vi "test_marcel.vi"() -> ()   [LabVIEW 2012]
uses:
  OLD_apparatus_VI/VI/Clearing_mode.ctl
  OLD_apparatus_VI/VI/Readout_mode.ctl
  OLD_apparatus_VI/VI/ADC_gain.ctl
  OLD_apparatus_VI/VI/Image_type.ctl
panel:
  out "Numeric":i32
  out "Data type":u32
  in  "Image type":T1=6 items=["8 bit signed"=1, "16 bit signed"=2, "32 bit signed"=3, "32 bit floating"=4, "64 bit floating"=5, "8 bit unsigned"=6, "16 bit unsigned"=7, "32 bit unsigned"=8]
  in  "Number of Images":u32=1000
  in  "Acquire / Focus Flag":u32=1
  in  "stop":bool=TRUE
  out "Number of Cameras":i32
  out "img":sgl[][](graph)
  out "Ydim":u32
  out "Xdim":u32
  out "Camera Handle":u32
  out "error out":errorcluster
  out "Image Handle":u32
  in  "ADC Gain":T2=-1 items=["Use current ADC"=-1, "Use the fastest ADC"=-2, "Use the slowest ADC"=-3]
  in  "ReadoutMode":T3=2.0 caption="Readout Mode" items=["Normal readout"=1.0, "Frame transfer readout"=2.0, "MPP readout"=3.0, "Frame transfer MPP"=4.0, "Alternate timing for normal readout"=5.0, "Alternate timing for frame transfer"=6.0, "Alternate timing for MPP"=7.0, "Alternate timing for frame transfer MPP"=8.0, "Interline"=9.0]
  in  "ClearMode":T4=1.0 caption="Clearing Mode" items=["Clear never"=1.0, "Clear pre-exposure"=2.0, "Clear pre-sequence"=3.0, "Clear post-sequence"=4.0, "Clear pre- and post-sequence"=5.0, "Clear pre-exposure and post-sequence"=6.0]
  in  "EMGain":dbl=3500.0 caption="EM Gain" format="%.2f"
  in  "Exposure (sec)":dbl=0.01 format="%.3f"
  in  "Temperature":dbl=-70.0 format="%.2f"
  in  "error in (no error)":errorcluster
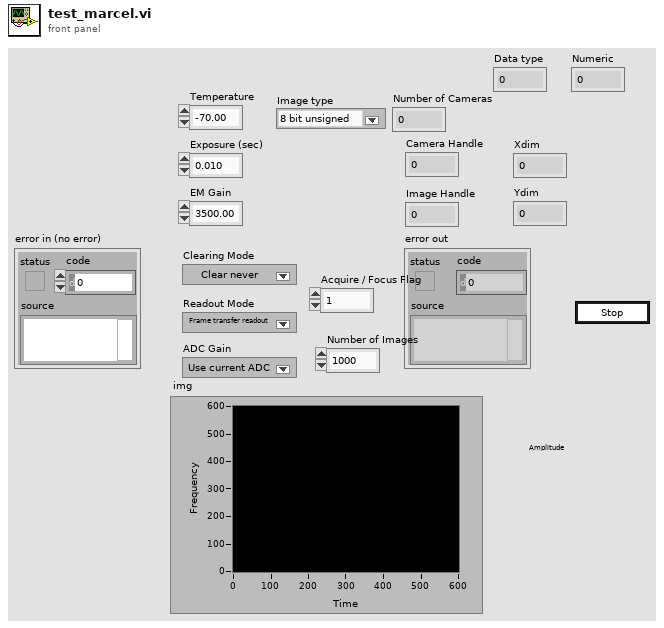
[diagram p1: front panel]
types:
  T1 = typedef "Image_type.ctl" = u32
  T2 = typedef "ADC_gain.ctl" = i32
  T3 = typedef "Readout_mode.ctl" = dbl
  T4 = typedef "Clearing_mode.ctl" = dbl
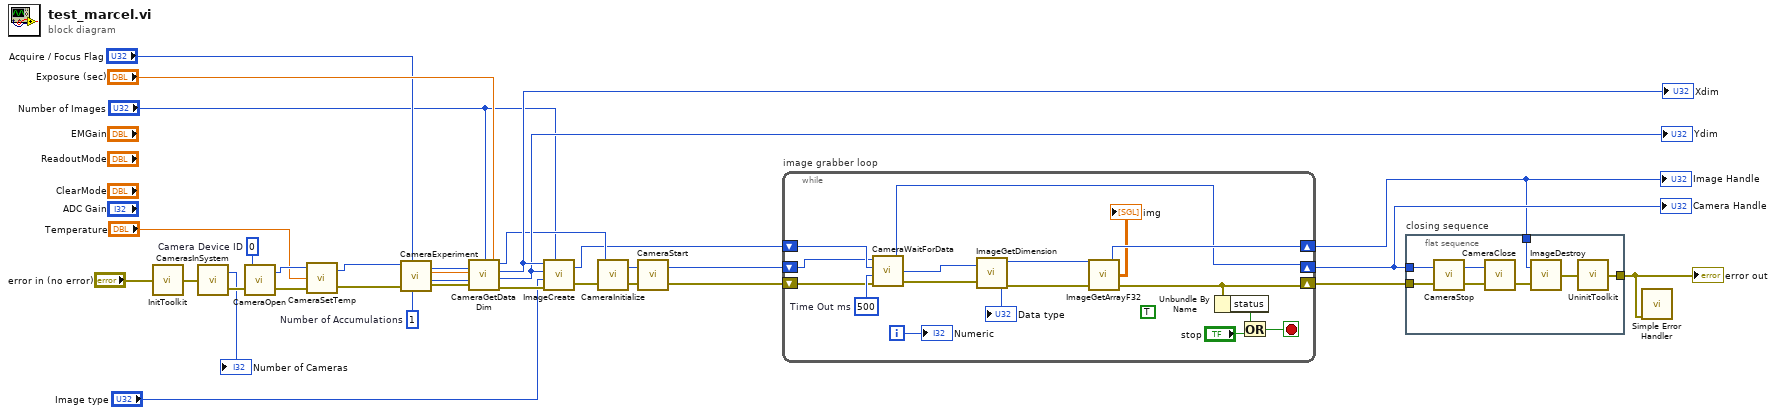
[diagram p0: block diagram]
diagram:
  w14 = u32 1  # Number of Accumulations
  w30 = u32 0  # Camera Device ID
  n1 = call <userlib>:"InitToolkit.vi"("error in"="error in (no error)") -> ("error out"=w6:errorcluster)
  n2 = call <userlib>:"CamerasInSystem.vi"("error in"=w6) -> ("Number of Cameras"=→"Number of Cameras":i32, "error out"=w18:errorcluster)
  n3 = call <userlib>:"CameraOpen.vi"("error in"=w18, "Camera Device ID"=w30) -> ("error out"=w28:errorcluster, "Camera Handle"=w29:u32)
  n4 = call <userlib>:"CameraSetTemp.vi"("error in (no error)"=w28, "Temperature"="Temperature", "Camera Handle"=w29) -> ("error out"=w2:errorcluster, "Camera Handle"=w1:u32)
  n5 = call <userlib>:"CameraExperiment.vi"("Number of Accumulations"=w14, "Acquire / Focus Flag"="Acquire / Focus Flag", "error in"=w2, "Number of Images"="Number of Images", "Exposure (sec)"="Exposure (sec)", "Camera Handle"=w1) -> ("error out"=w26:errorcluster, "Camera Handle"=w10:u32)
  n6 = call <userlib>:"CameraGetDataDim.vi"("Camera Handle"=w10, "error in"=w26) -> ("Camera Handle"=w9:u32, "Xdim"=w23:u32, "Ydim"=w22:u32, "error out"=w24:errorcluster)
  "Xdim" <- w23
  "Ydim" <- w22
  n7 = call <userlib>:"ImageCreate.vi"("X dimension"=w23, "Y dimension"=w22, "Data Type"="Image type", "error in"=w24, "Number Of Frames"="Number of Images") -> ("Image Handle"=w5:u32, "error out"=w12:errorcluster)
  n8 = call <userlib>:"CameraInitialize.vi"("error in"=w12, "Camera Handle"=w9) -> ("error out"=w11:errorcluster, "Camera Handle"=w13:u32)
  n9 = call <userlib>:"CameraStart.vi"("error in"=w11, "Camera Handle"=w13) -> ("error out"=w4:errorcluster, "Camera Handle"=w3:u32)
  n10 = while "image grabber loop" {
    shift-right: [w47] -> w20
    shift-left: w5 -> [w46]
    shift-right: [w38] -> w21
    shift-left: w3 -> [w33]
    shift-right: [w48] -> w19
    shift-left: w4 -> [w34]
    i -> [w32]
    stop <- w44 stop-if-true
    w41 = u32 500  # Time Out ms
    (unwired) TRUE
    n11 = call <userlib>:"CameraWaitForData.vi"("error in"=w34, "Time Out ms"=w41, "Image Handle"=w46, "Camera Handle"=w33) -> ("error out"=w36:errorcluster, "Image Handle"=w37:u32, "Camera Handle"=w38:u32)
    n12 = call <userlib>:"ImageGetDimension.vi"("Image Handle"=w37, "error in"=w36) -> ("Data type"=→"Data type":u32, "Image Handle"=w35:u32, "error out"=w40:errorcluster)  [unwired: 3 out]
    n13 = call <userlib>:"ImageGetArrayF32.vi"("error in"=w40, "Image Handle"=w35) -> ("error out"=w48:errorcluster, "Array Float 32"=→"img":sgl[][], "Image Handle"=w47:u32)  [unwired: 1 in]
    n14 = Unbundle By Name(w48) -> ("status"=w45:bool)
    n15 = Or(x=w45, y="stop") -> (x .or. y?=w44:bool)
    "Numeric" <- w32
  }
  "Image Handle" <- w20
  "Camera Handle" <- w21
  n16 = flat-sequence "closing sequence" {
    tunnel: w21 -> [w50]
    tunnel: w20 -> [w54]
    tunnel: w19 -> [w52]
    tunnel: [w53] -> w16
    frame #0 {
      n17 = call <userlib>:"CameraStop.vi"("error in"=w52, "Camera Handle"=w50) -> ("error out"=w51:errorcluster, "Camera Handle"=w49:u32)
      n18 = call <userlib>:"CameraClose.vi"("error in"=w51, "Camera Handle"=w49) -> ("error out"=w55:errorcluster)
      n19 = call <userlib>:"ImageDestroy.vi"("error in"=w55, "Data handle"=w54) -> ("error out"=w56:errorcluster)
      n20 = call <userlib>:"UninitToolkit.vi"("error in"=w56) -> ("error out"=w53:errorcluster)
    }
  }
  n21 = call <vilib>:"Simple Error Handler.vi"("error in (no error)"=w16) -> ()  [unwired: 4 in, 5 out]
  "error out" <- w16
